vi "Write UIEvent.vi"(8 "Error In":errorcluster, 10 "Event ID":T1, 11 "GEA2 Reference In":refnum<k24>) -> (0 "Error Out":errorcluster, 3 "GEA2 Reference Out":refnum<k24>)   [LabVIEW 2016, in "Centauro.lvlib"]
uses:
  Projects/Centauro.lvlib
  Q:/Common/DLLs/GEA3/GeaCommunication.dll
  Common/DLLs/GEA3/GeaCommunication.dll
  Tools/Laundry/Centauro Tool/Centauro Tool Support/type defs/Event Sequence.ctl
  Common/LabVIEW GEA2 Toolkit/LabVIEW_GEA2_Toolkit.lvlibp/type defs/Source_Destination.ctl
  Common/LabVIEW GEA2 Toolkit/LabVIEW_GEA2_Toolkit.lvlibp/type defs/ERD Read Data In.ctl
  Common/LabVIEW GEA2 Toolkit/LabVIEW_GEA2_Toolkit.lvlibp/type defs/Data Type.ctl
  Common/LabVIEW GEA2 Toolkit/LabVIEW_GEA2_Toolkit.lvlibp
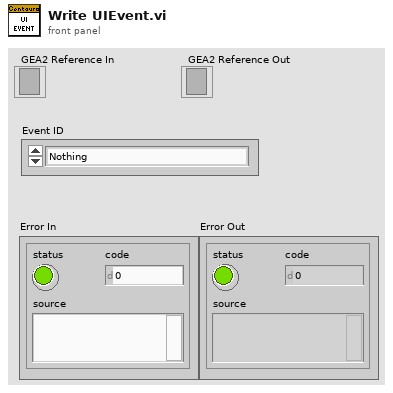
[diagram p1: front panel]
types:
  T1 = typedef "Event Sequence.ctl" = enum16{"Nothing", "StartButtonPress", "StartButtonRelease", "DeepRinseKeyPress", "DeepRinseKeyRelease", "CycleKnobPosition0", "CycleKnobPosition1", "CycleKnobPosition2", "CycleKnobPosition3", "CycleKnobPosition4", "CycleKnobPosition5", "CycleKnobPosition6", "CycleKnobPosition7", "CycleKnobPosition8", "CycleKnobPosition9", "CycleKnobPosition10", "CycleKnobPosition11", "OptionKnob1Position0", "OptionKnob1Position1", "OptionKnob1Position2", "OptionKnob1Position3", "OptionKnob1Position4", "OptionKnob1Position5", "OptionKnob2Position0", "OptionKnob2Position1", "OptionKnob2Position2", "OptionKnob2Position3", "OptionKnob2Position4"}
  T2 = typedef "LabVIEW_GEA2_Toolkit.lvlibp/ERD Read Data In.ctl" = cluster{"ERD Number":u16, "Data Type":T3}
  T3 = typedef "LabVIEW_GEA2_Toolkit.lvlibp/Data Type.ctl" = enum16{"string", "boolean", "uint8_t", "uint16_t", "uint32_t", "uint64_t", "int8_t", "int16_t", "int32_t", "int64_t"}
  T4 = typedef "LabVIEW_GEA2_Toolkit.lvlibp/Source_Destination.ctl" = cluster{"Source":u8, "Destination":u8}
  T5 = typedef "LabVIEW_GEA2_Toolkit.lvlibp/ERD Read Data Out.ctl" = cluster{"ERD Number":u16, "Data":string}
  T6 = typedef "LabVIEW_GEA2_Toolkit.lvlibp/ERD Write Data In.ctl" = cluster{"ERD Number":u16, "Data Type":T3, "Data":string}
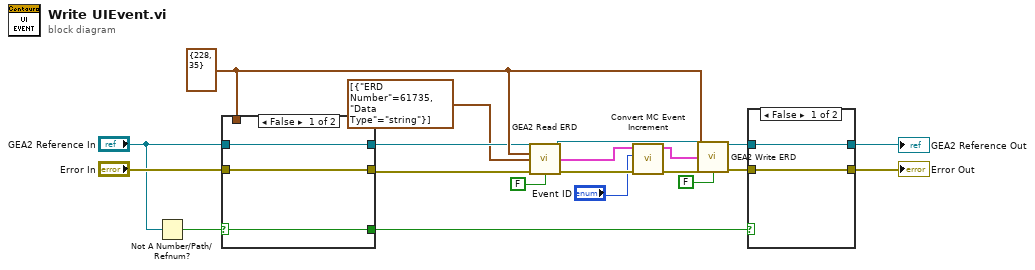
[diagram p0: block diagram]
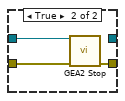
[diagram p2: hidden frame]
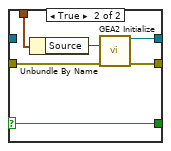
[diagram p3: hidden frame]
diagram:
  w13 = T4 {"Source"=228, "Destination"=35} ("GEA Inputs")
  n1 = Not A Number/Path/Refnum?(number/path/refnum="GEA2 Reference In") -> (NaN/Path/Refnum?=w15:bool)
  n2 = case shown="False" w15 {
    selector: w15 -> [w21 w24]
    tunnel: "Error In" -> [w22 w29]
    tunnel: [w22 w28] -> w10
    tunnel: "GEA2 Reference In" -> [w23 _]
    tunnel: [w23 w27] -> w12
    tunnel: w13 -> [_ w25]
    tunnel: [w21 w24] -> w5
    frame False {
    }
    frame True {
      n3 = Unbundle By Name(w25) -> ("Source"=w26:u8)
      n4 = call "GEA2 Initialize.vi"("Source Address"=w26, "error in"=w29) -> ("GEA2 Reference Out"=w27:refnum<k24>, "error out"=w28:errorcluster)  [unwired: 11 in, 1 out]
    }
  }
  n5 = call "GEA2 Read ERD.vi"("GEA2 Reference In"=w12, "GEA Inputs"=w13, "Read ERD List"=T2[] [{"ERD Number"=61735, "Data Type"=enum."string"}], "Error In"=w10, "Verify ERD Response?"=FALSE) -> ("GEA2 Reference Out"=w11:refnum<k24>, "ERD Data Out"=w8:T5[], "Error Out"=w7:errorcluster)  [unwired: 7 in, 1 out]
  n6 = call "Convert MC Event Increment.vi"("error in (no error)"=w7, "Event ID"="Event ID", "ERD Data In"=w8) -> ("error out"=w6:errorcluster, "Send ERD Data"=w14:T6[])  [unwired: 7 in]
  n7 = call "GEA2 Write ERD.vi"("GEA2 Reference In"=w11, "GEA Inputs"=w13, "Write ERD List"=w14, "Error In"=w6, "Verify ERD Response?"=FALSE) -> ("GEA2 Reference Out"=w17:refnum<k24>, "Error Out"=w3:errorcluster)  [unwired: 8 in, 1 out]
  n8 = case shown="False" w5 {
    tunnel: [w30 w34] -> w19
    tunnel: w17 -> [w31 w33]
    tunnel: [w31 _] -> w18
    tunnel: w3 -> [w30 w32]
    frame False {
    }
    frame True {
      n9 = call "GEA2 Stop.vi"("GEA2 Reference In"=w33, "Error In"=w32) -> ("Error Out"=w34:errorcluster)  [unwired: 13 in]
    }
  }
  "Error Out" <- w19
  "GEA2 Reference Out" <- w18
